vi "Set error.vi"(8 "error in (no error)":errorcluster, 11 "Control-Server in":refnum<class "Control-Server.lvclass">) -> (0 "error out":errorcluster, 3 "Control-Server out":refnum<class "Control-Server.lvclass">)   [LabVIEW 2018, in "Control-Server.lvclass"]
uses:
  Control-Server.lvclass
  C:/Users/Sergey Denisov/Documents/REPS/TRANCON/Classes/GeneralFunctionality/GeneralFunctionality.lvclass
  GeneralFunctionality/GeneralFunctionality.lvclass/GeneralFunctionality.ctl
  GeneralFunctionality/GeneralFunctionality.lvclass
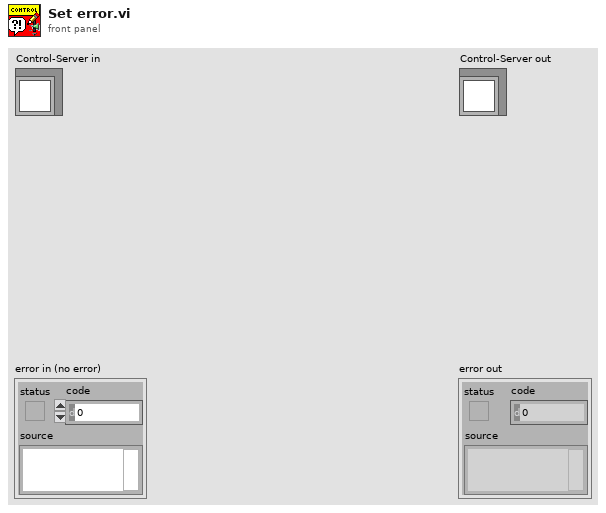
[diagram p1: front panel]
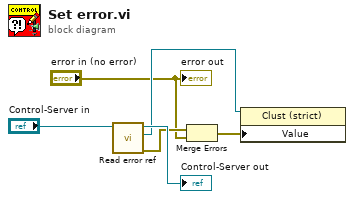
[diagram p0: block diagram]
diagram:
  n1 = call "Read error ref.vi"("GeneralFunctionality in"="Control-Server in") -> ("error out"=w3:errorcluster, "error"=w4:refnum<vi>, "GeneralFunctionality out"=→"Control-Server out":refnum<class "Control-Server.lvclass">)  [unwired: 8 in]
  n2 = Merge Errors(w3, "error in (no error)") -> (w1:errorcluster)
  n3 = property class="Clust (strict)"(reference=w4, "Value"=w1) -> ()  [unwired: 1 in, 2 out]
  "error out" <- "error in (no error)"
